vi "Remove Item.vi"(8 "error in (no error)":errorcluster, 10 "Item":refnum<class "Item.lvclass">, 11 "Listbox in":refnum<class "Listbox.lvclass">) -> (0 "error out":errorcluster, 3 "Listbox out":refnum<class "Listbox.lvclass">)   [LabVIEW 2016, in "Listbox.lvclass"]
uses:
  Listbox.lvclass
  Interfaces/Item/Item.lvclass
  Listbox Item/Listbox Item.lvclass
  Listbox.lvclass/Listbox.ctl
  Listbox Item/Listbox Item.lvclass/Listbox Item.ctl
  <vilib>/Utility/error.llb/Error Cluster From Error Code.vi
  <vilib>/ErrorRing/Error Ring.xnode
panel:
  # "NOTICE -- YOU MUST LEAVE THIS NOTICE IN PLACE.\n\nCopyright (c) 2017, LIANG LIU Shawn.Liu.cn@gmail.com\nAll rights reserved.\n\nRedistribution and use in source and binary forms, with or without modification, are permitted provided that the following conditions are met:\n-Redistributions of source code must retain the above copyright notice, this list of conditions and the following disclaimer.\n-Redistributions in binary form must reproduce the above copyright notice, this list of conditions and the following disclaimer in the documentation and/or other materials provided with the distribution.\n-Neither the name of the eLp nor the names of its contributors may be used to endorse or promote products derived from this software without specific prior written permission.\n\nTHIS SOFTWARE IS PROVIDED BY THE COPYRIGHT HOLDERS AND CONTRIBUTORS \"AS IS\" AND ANY EXPRESS OR IMPLIED WARRANTIES, INCLUDING, BUT NOT LIMITED TO, THE IMPLIED WARRANTIES OF MERCHANTABILITY AND FITNESS FOR A PARTICULAR PURPOSE ARE DISCLAIMED. IN NO EVENT SHALL THE COPYRIGHT HOLDER OR CONTRIBUTORS BE LIABLE FOR ANY DIRECT, INDIRECT, INCIDENTAL, SPECIAL, EXEMPLARY, OR CONSEQUENTIAL DAMAGES (INCLUDING, BUT NOT LIMITED TO, PROCUREMENT OF SUBSTITUTE GOODS OR SERVICES; LOSS OF USE, DATA, OR PROFITS; OR BUSINESS INTERRUPTION) HOWEVER CAUSED AND ON ANY THEORY OF LIABILITY, WHETHER IN CONTRACT, STRICT LIABILITY, OR TORT (INCLUDING NEGLIGENCE OR OTHERWISE) ARISING IN ANY WAY OUT OF THE USE OF THIS SOFTWARE, EVEN IF ADVISED OF THE POSSIBILITY OF SUCH DAMAGE."
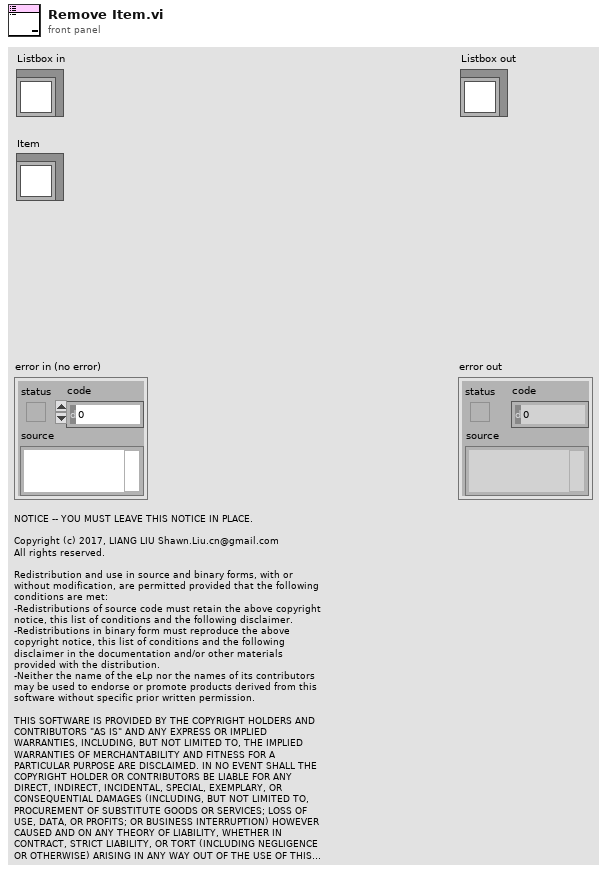
[diagram p1: front panel]
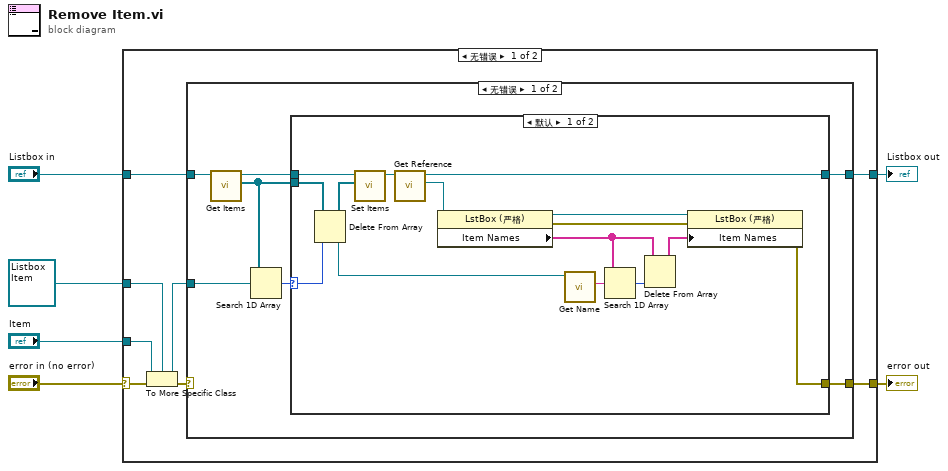
[diagram p0: block diagram]
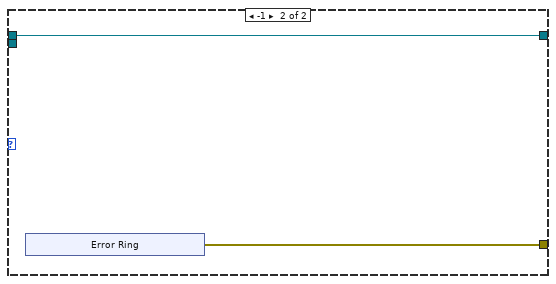
[diagram p2: hidden frame]
diagram:
  n1 = case shown="无错误" "error in (no error)" {
    selector: "error in (no error)" -> [w10 w46]
    tunnel: refnum<class "Listbox Item.lvclass"> refnum ("Listbox Item.lvclass") -> [w14 _]
    tunnel: "Listbox in" -> [w13 w45]
    tunnel: [w12 w45] -> w4
    tunnel: "Item" -> [w11 _]
    tunnel: [w9 w46] -> w1
    frame No Error {
      n2 = To More Specific Class(target class=w14, reference=w11, error in=w10) -> (specific class reference=w8:refnum<class "Listbox Item.lvclass">, error out=w7:errorcluster)
      n3 = case shown="无错误" w7 {
        selector: w7 -> [_ w44]
        tunnel: w13 -> [w21 w43]
        tunnel: [w20 w43] -> w12
        tunnel: [w19 w44] -> w9
        tunnel: w8 -> [w18 _]
        frame No Error {
          n4 = call "Get Items.vi"("Listbox in"=w21) -> ("Items"=w16:refnum<class "Listbox Item.lvclass">[], "Listbox out"=w17:refnum<class "Listbox.lvclass">)  [unwired: 9 in]
          n5 = Search 1D Array(1D array=w16, element=w18) -> (index of element=w15:i32)  [unwired: 1 in]
          n6 = case shown="默认" w15 {
            selector: w15 -> [w22 _]
            tunnel: [w36 w38] -> w20
            tunnel: [w35 w37] -> w19
            tunnel: w17 -> [w34 w38]
            tunnel: w16 -> [w33 _]
            frame Default {
              n7 = Delete From Array(array=w33, index=w22) -> (deleted portion=w24:refnum<class "Listbox Item.lvclass">, array with subset deleted=w25:refnum<class "Listbox Item.lvclass">[])  [unwired: 1 in]
              n8 = call "Set Items.vi"("Items"=w25, "Listbox in"=w34) -> ("Listbox out"=w29:refnum<class "Listbox.lvclass">)  [unwired: 9 in]
              n9 = call "Get Reference.vi"("Listbox in"=w29) -> ("Reference"=w31:refnum<vi>, "Listbox out"=w36:refnum<class "Listbox.lvclass">)  [unwired: 9 in]
              n10 = property class="LstBox (严格)"(reference=w31) -> (reference out=w32:refnum<vi>, error out=w30:errorcluster, "Item Names"=w26:string[])  [unwired: 1 in]
              n11 = call "Get Name.vi"("Listbox Item in"=w24) -> ("Name"=w23:string)  [unwired: 9 in, 1 out]
              n12 = Search 1D Array(1D array=w26, element=w23) -> (index of element=w27:i32)  [unwired: 1 in]
              n13 = Delete From Array(array=w26, index=w27) -> (array with subset deleted=w28:string[])  [unwired: 1 in, 1 out]
              n14 = property class="LstBox (严格)"(reference=w32, error in=w30, "Item Names"=w28) -> (error out=w35:errorcluster)  [unwired: 1 out]
            }
            frame -1 {
              n15 = xnode "Error Ring"() -> ("错误输出"=w37:errorcluster)
            }
          }
        }
        frame Error {
        }
      }
    }
    frame Error {
    }
  }
  "error out" <- w1
  "Listbox out" <- w4
